vi "Loop_Timing.vi"(8 "error in":errorcluster, 10 "Outer Loop sample rate in":dbl=20.0, 11 "IMU_sample_rate in":i32=200) -> (0 "error out":errorcluster, 1 "Outer Loop Start":bool, 2 "30hz Start":bool, 3 "Hz":dbl format="%#_4g")   [LabVIEW 2014]
panel:
  in  "IMU_sample_rate":i32=200
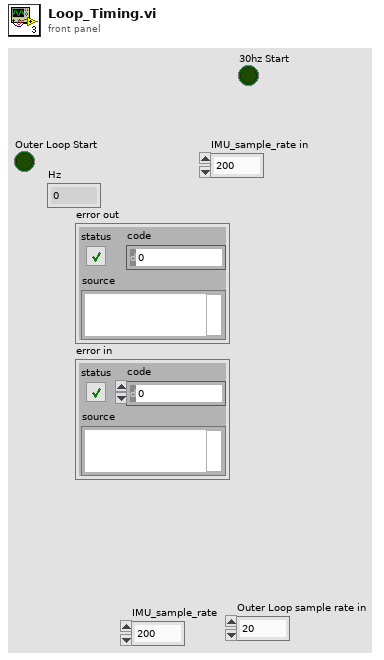
[diagram p1: front panel]
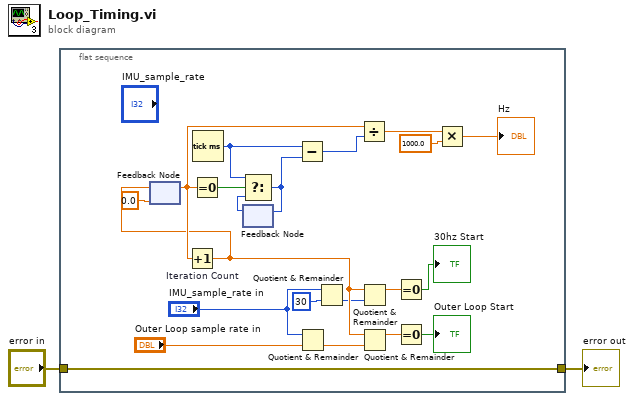
[diagram p0: block diagram]
diagram:
  n1 = flat-sequence {
    tunnel: "error in" -> [w13]
    tunnel: [w13] -> w1
    frame #0 {
      n2 = feedback #1(0.0) -> (w19:dbl)
      n3 = Increment "Iteration Count"(x=w19) -> (x+1=w6:dbl)
      n4 = feedback-in #1(w6) -> ()
      n5 = Equal To 0?(x=w19) -> (x = 0?=w18:bool)
      n6 = Tick Count (ms)() -> (millisecond timer value=w17:u32)
      n7 = feedback #2() -> (w16:u32)  [unwired: 1 in]
      n8 = Select(t=w17, s=w18, f=w16) -> (s? t:f=w15:u32)
      n9 = feedback-in #2(w15) -> ()
      n10 = Subtract(x=w17, y=w15) -> (x-y=w14:u32)
      n11 = Quotient & Remainder(x="IMU_sample_rate in", y="Outer Loop sample rate in") -> (floor(x/y)=w10:dbl)  [unwired: 1 out]
      n12 = Quotient & Remainder(x="IMU_sample_rate in", y=30) -> (floor(x/y)=w3:i32)  [unwired: 1 out]
      n13 = Divide(x=w19, y=w14) -> (x/y=w22:dbl)
      n14 = Quotient & Remainder(x=w6, y=w3) -> (x-y*floor(x/y)=w5:dbl)  [unwired: 1 out]
      n15 = Quotient & Remainder(x=w6, y=w10) -> (x-y*floor(x/y)=w12:dbl)  [unwired: 1 out]
      n16 = Equal To 0?(x=w5) -> (x = 0?=→"30hz Start":bool)
      n17 = Equal To 0?(x=w12) -> (x = 0?=→"Outer Loop Start":bool)
      n18 = Multiply(x=w22, y=1000.0) -> (x*y=→"Hz":dbl)
    }
  }
  "error out" <- w1
